vi "UnlockECU.SendSeedToWindowsAndWaitOnKey.vi"(7 "Addon Name":string, 8 "error in (no error)":errorcluster, 9 "Security":T3={"Type"=enum."None", "Source DLL Path"=path "", "Target DLL Path"=path "", "Security Level"=1, "Static Master Key"="", "Max Key Length"=1, "Host IP Address"="", "ECU  Variant"=0, "Optional Parameter"=0}, 10 "Seed":u8[](array[numeric]), 11 "TCP Info":T1) -> (0 "error out":errorcluster, 2 "Error code":i32, 3 "Key":u8[](array[numeric]))   [LabVIEW 2019, in "Diagnostics Addon Engine.lvlib"]
uses:
  Diagnostics Addon Engine.lvlib
  Addon Shared/Types/Security.ctl
  Addon Shared/Types/Security.Type.ctl
  <vilib>/NI/STM/TCP/TCP Connection Info.ctl
  Service/Service Shared/UnlockECU.SendSeedToWindowsAndWaitOnKeyCmd.ctl
  Service/Service Shared/UnlockECU.SendSeedToWindowsAndWaitOnKeyResp.ctl
  <vilib>/NI/STM/TCP/Get Connection Reference (TCP).vi
  <vilib>/NI/NI VeriStand Addon Network Comm/Shared/NI VeriStand Addon Network Comm Shared.lvlib
  <vilib>/NI/STM/NI STM.lvlib
  Service/Service Shared/Diagnostic Unlock ECU Service Shared.lvlib
  Addon Shared/Diagnostics Addon Shared.lvlib
  <vilib>/NI/STM/SubVIs/MetaDataElement.ctl
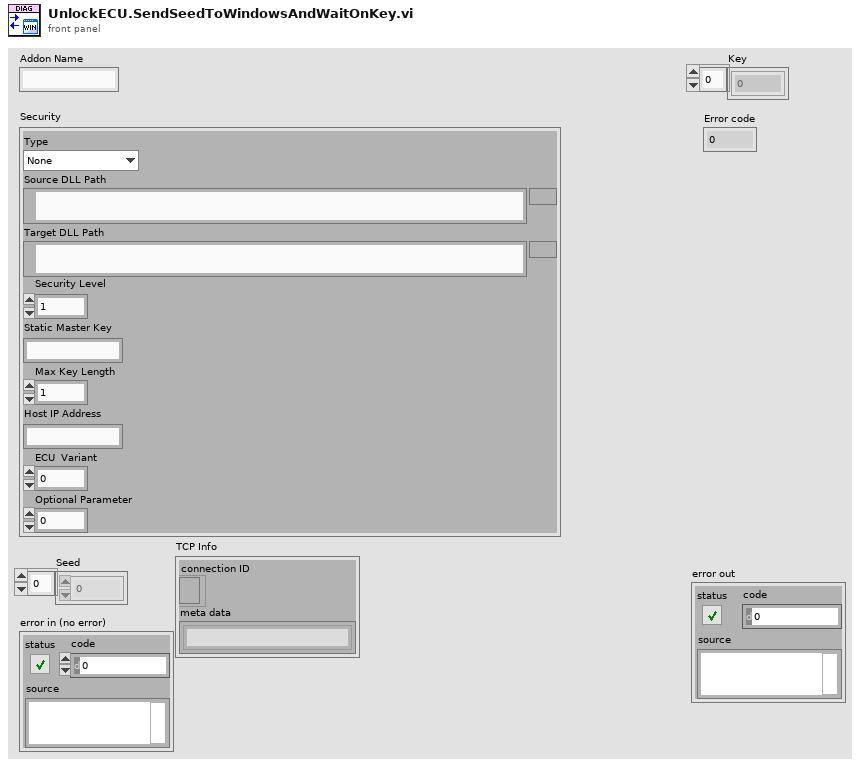
[diagram p1: front panel]
types:
  T1 = typedef "NI STM.lvlib/TCP Connection Info.ctl" = cluster{"connection ID":refnum<k5>, "meta data":T2[]}
  T2 = typedef "NI STM.lvlib/MetaDataElement.ctl" = string
  T3 = typedef "Diagnostics Addon Shared.lvlib/Security.ctl" = cluster{"Type":T4, "Source DLL Path":path, "Target DLL Path":path, "Security Level":u32, "Static Master Key":string, "Max Key Length":u32, "Host IP Address":string, "ECU  Variant":i8, "Optional Parameter":i8}
  T4 = typedef "Diagnostics Addon Shared.lvlib/Security.Type.ctl" = enum16{"None", "SeedKey DLL", "MasterKey (Channel)", "MasterKey (Static)", "SeedKey DLL (Windows)"}
  T5 = typedef "Diagnostic Unlock ECU Service Shared.lvlib/UnlockECU.SendSeedToWindowsAndWaitOnKeyCmd.ctl" = cluster{"Source DLL Path":path, "Security Level":u32, "Max Key Length":u32, "Seed":u8[], "ECU  Variant":i8, "Addon Name":string, "Optional Parameter":i8}
  T6 = typedef "Diagnostic Unlock ECU Service Shared.lvlib/UnlockECU.SendSeedToWindowsAndWaitOnKeyResp.ctl" = cluster{"DLL Error":errorcluster, "Key Length":u32, "Key":u8[]}
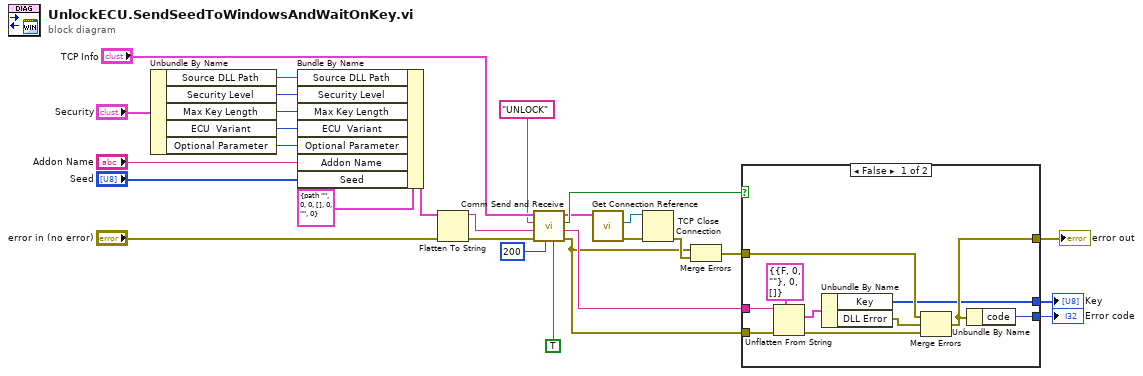
[diagram p0: block diagram]
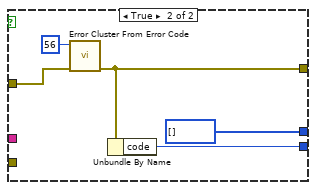
[diagram p2: hidden frame]
diagram:
  n1 = Unbundle By Name("Security") -> ("Source DLL Path"=w13:path, "Security Level"=w12:u32, "Max Key Length"=w11:u32, "ECU  Variant"=w10:i8, "Optional Parameter"=w9:i8)
  n2 = Bundle By Name(cluster=T5 {"Source DLL Path"=path "", "Security Level"=0, "Max Key Length"=0, "Seed"=[], "ECU  Variant"=0, "Addon Name"="", "Optional Parameter"=0}, "Source DLL Path"=w13, "Security Level"=w12, "Max Key Length"=w11, "ECU  Variant"=w10, "Optional Parameter"=w9, "Addon Name"="Addon Name", "Seed"="Seed") -> (w15:T5)
  n3 = Flatten To String(anything=w15, error in (no error)="error in (no error)") -> (data string=w5:string, error out=w7:errorcluster)  [unwired: 2 in, 1 out]
  n4 = call <vilib>:"Comm Send and Receive.vi"("Resp Required?"=TRUE, "Timeout (ms)"=u32 200, "error in (no error)"=w7, "Data"=w5, "Name"="UNLOCK", "connection info"="TCP Info") -> ("error out"=w3:errorcluster, "Data"=w8:string, "Timed Out?"=w20:bool, "connection info"=w18:T1)  [unwired: 2 in]
  n5 = call-poly <vilib>:"Get Connection Reference.vi"("connection info in"=w18) -> ("error out"=w2:errorcluster, "connection ID out"=w19:refnum<k5>)  [unwired: 8 in, 1 out]
  n6 = TCP Close Connection(connection ID=w19, error in (no error)=w2) -> (error out=w4:errorcluster)  [unwired: 1 in, 1 out]
  n7 = Merge Errors(w3, w4) -> (w1:errorcluster)
  n8 = case shown="False" w20 {
    tunnel: w1 -> [w32 w42]
    tunnel: [w31 w41] -> w24
    tunnel: w3 -> [w34 _]
    tunnel: w8 -> [w33 _]
    tunnel: [w30 w40] -> w23
    tunnel: [w29 u8[] [] ("Key")] -> w22
    frame False {
      n9 = Unflatten From String(type=T6 {"DLL Error"={"status"=FALSE, "code"=0, "source"=""}, "Key Length"=0, "Key"=[]}, binary string=w33, error in (no error)=w34) -> (value=w37:T6, error out=w35:errorcluster)  [unwired: 2 in, 1 out]
      n10 = Unbundle By Name(w37) -> ("Key"=w29:u8[], "DLL Error"=w38:errorcluster)
      n11 = Merge Errors(w32, w38, w35) -> (w31:errorcluster)
      n12 = Unbundle By Name(w31) -> ("code"=w30:i32)
    }
    frame True {
      n13 = call <vilib>:"Error Cluster From Error Code.vi"("error in (no error)"=w42, "error code (0)"=56 ("code")) -> ("error out"=w41:errorcluster)  [unwired: 7 in]
      n14 = Unbundle By Name(w41) -> ("code"=w40:i32)
    }
  }
  "error out" <- w24
  "Key" <- w22
  "Error code" <- w23
